vi "Set Output Values.vi"(8 "error in (no error)":errorcluster, 11 "Spectrum Recorder in":refnum<class "Spectrum Recorder.lvclass">) -> (0 "error out":errorcluster, 3 "Spectrum Recorder out":refnum<class "Spectrum Recorder.lvclass">)   [LabVIEW 2016, in "Spectrum Recorder.lvclass"]
uses:
  Spectrum Recorder.lvclass
  Spectrum Recorder.lvclass/Spectrum Recorder.ctl
  Read Spectrum Recorder Configuration.vi
  NHMFL_Core/Libraries/Red Pitaya/RP Core/RP Transceiver/RP Transceiver.lvclass
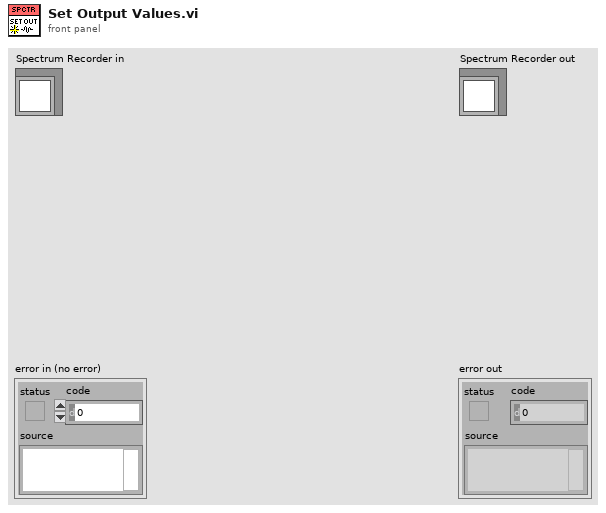
[diagram p1: front panel]
types:
  T1 = typedef "Spectrum Recorder Configuration.ctl" = cluster{"Start":dbl, "End":dbl, "Duration":dbl, "Filter time constant":dbl, "Repeat (-1: forever)":i32, "Update rate":dbl, "Data storage folder":path}
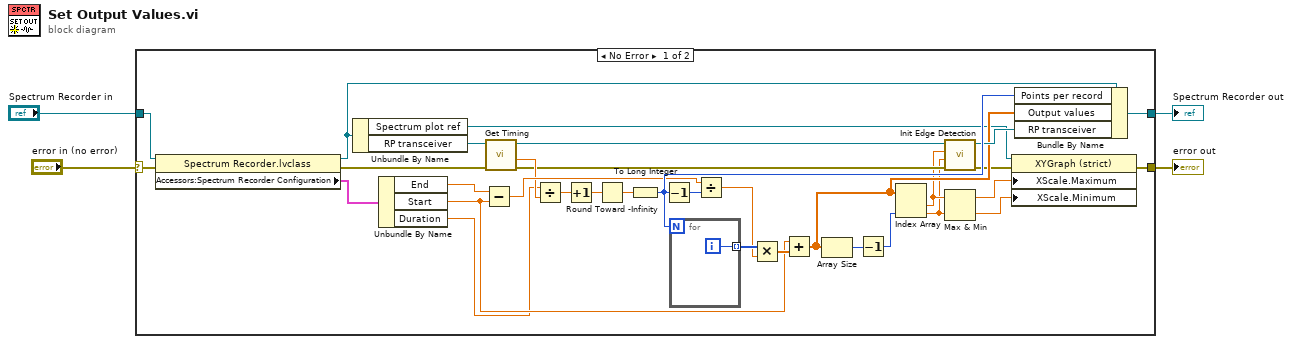
[diagram p0: block diagram]
diagram:
  n1 = case shown="No Error" "error in (no error)" {
    selector: "error in (no error)" -> [w8 w40]
    tunnel: [w19 w40] -> w3
    tunnel: [w27 w39] -> w1
    tunnel: "Spectrum Recorder in" -> [w11 w39]
    frame No Error {
      n2 = property class="Spectrum Recorder.lvclass"(reference=w11, error in=w8) -> (reference out=w10:refnum<class "Spectrum Recorder.lvclass">, error out=w9:errorcluster, "Accessors:Spectrum Recorder Configuration"=w12:T1)
      n3 = Unbundle By Name(w10) -> ("Spectrum plot ref"=w20:refnum<vi>, "RP transceiver"=w13:refnum<class "RP Transceiver.lvclass">)
      n4 = Unbundle By Name(w12) -> ("End"=w7:dbl, "Start"=w6:dbl, "Duration"=w5:dbl)
      n5 = Subtract(x=w7, y=w6) -> (x-y=w33:dbl)
      n6 = call-dynamic "Get Timing.vi"("error in (no error)"=w9, "RP Transceiver in"=w13) -> ("error out"=w26:errorcluster, "dt"=w28:dbl, "RP Transceiver out"=w24:refnum<class "RP Transceiver.lvclass">)  [unwired: 5 in, 2 out]
      n7 = Divide(x=w5, y=w28) -> (x/y=w31:dbl)
      n8 = Increment(x=w31) -> (x+1=w30:dbl)
      n9 = Round Toward -Infinity(1:w30) -> (0:w29:dbl)
      n10 = To Long Integer(number=w29) -> (32bit integer=w34:i32)
      n11 = Decrement(x=w34) -> (x-1=w32:i32)
      n12 = for {
        N: w34 -> [_]
        tunnel: [w38] -> w36 mode=indexing
        i -> [w38]
      }
      n13 = Divide(x=w33, y=w32) -> (x/y=w35:dbl)
      n14 = Multiply(x=w36, y=w35) -> (x*y=w37:dbl[])
      n15 = Add(x=w6, y=w37) -> (x+y=w23:dbl[])
      n16 = Array Size(array=w23) -> (size(s)=w22:i32)
      n17 = Decrement(x=w22) -> (x-1=w21:i32)
      n18 = Index Array(array=w23, index #2=w21) -> (element #1=w17:dbl, element #2=w16:dbl)  [unwired: 1 in]
      n19 = call-dynamic "Init Edge Detection.vi"("error in (no error)"=w26, "Last output"=w16, "First output"=w17, "RP Transceiver in"=w24) -> ("error out"=w18:errorcluster, "RP Transceiver out"=w25:refnum<class "RP Transceiver.lvclass">)  [unwired: 6 in]
      n20 = Max & Min(x=w17, y=w16) -> (max(x,y)=w15:dbl, min(x,y)=w14:dbl)
      n21 = property class="XYGraph (strict)"(reference=w20, error in=w18, "XScale.Maximum"=w15, "XScale.Minimum"=w14) -> (error out=w19:errorcluster)  [unwired: 1 out]
      n22 = Bundle By Name(cluster=w10, "Points per record"=w34, "Output values"=w23, "RP transceiver"=w25) -> (w27:refnum<class "Spectrum Recorder.lvclass">)
    }
    frame Error {
    }
  }
  "error out" <- w3
  "Spectrum Recorder out" <- w1
